vi "Emballage_BDD_config_vue_onglet.vi"(8 "entrée d'erreur (pas d'erreur)":errorcluster, 10 "onglet_Actif":i32, 11 "TabControl en entrée":refnum<vi>) -> (0 "sortie d'erreur":errorcluster)   [LabVIEW 2020]
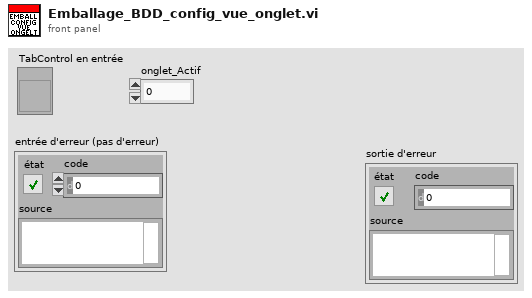
[diagram p1: front panel]
types:
  T1 = enum32{"Page Enabled", "Page Disabled", "Page Disabled & Grayed"}
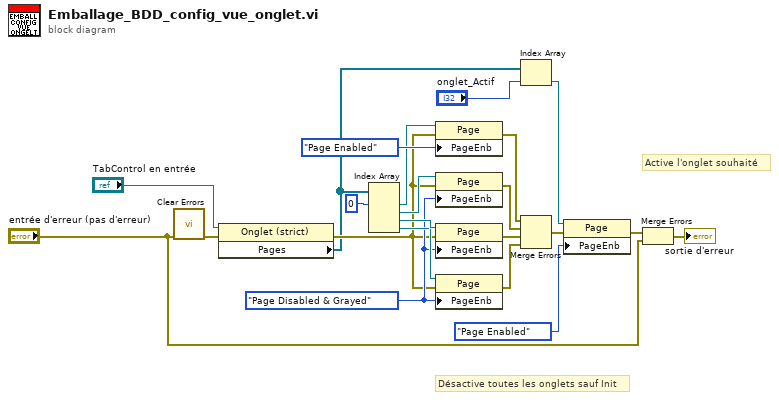
[diagram p0: block diagram]
diagram:
  w15 = T1."Page Disabled & Grayed" ("État d'activation de la page")
  # "Active l'onglet souhaité"
  # "Désactive toutes les onglets sauf Init"
  n1 = call <vilib>:"Clear Errors.vi"("error in (no error)"="entrée d'erreur (pas d'erreur)") -> ("error out"=w1:errorcluster)  [unwired: 5 in, 1 out]
  n2 = property on="Nœud de propriété" class="Onglet (strict)"(reference="TabControl en entrée", error in=w1) -> (error out=w14:errorcluster, "Pages"=w13:refnum<vi>[])  [unwired: 1 out]
  n3 = Index Array(array=w13, index #1=0 ("indice")) -> (element #1=w21:refnum<vi>, element #2=w18:refnum<vi>, element #3=w17:refnum<vi>, element #4=w16:refnum<vi>)  [unwired: 3 in]
  n4 = property class="Page"(reference=w21, error in=w14, "PageEnb"=T1."Page Enabled" ("État d'activation de la page")) -> (error out=w9:errorcluster)  [unwired: 1 out]
  n5 = property class="Page"(reference=w18, error in=w14, "PageEnb"=w15) -> (error out=w8:errorcluster)  [unwired: 1 out]
  n6 = property class="Page"(reference=w17, error in=w14, "PageEnb"=w15) -> (error out=w7:errorcluster)  [unwired: 1 out]
  n7 = property class="Page"(reference=w16, error in=w14, "PageEnb"=w15) -> (error out=w6:errorcluster)  [unwired: 1 out]
  n8 = Index Array(array=w13, index="onglet_Actif") -> (element=w11:refnum<vi>)
  n9 = Merge Errors(w9, w8, w7, w6) -> (w10:errorcluster)
  n10 = property class="Page"(reference=w11, error in=w10, "PageEnb"=T1."Page Enabled" ("État d'activation de la page")) -> (error out=w4:errorcluster)  [unwired: 1 out]
  n11 = Merge Errors(w4, "entrée d'erreur (pas d'erreur)") -> (→"sortie d'erreur":errorcluster)
